vi "Plot_Uniform_Array.vi"(10 "Top Left Building Centre":sgl[](array[numeric])=[-1400.0, -945.0, 50.0] format="%#.2f") -> (0 "Status":T2)   [LabVIEW 2015]
uses:
  Anemometry Sub Vis/Gen Trav/Multi_Run_Status.ctl
  Anemometry Sub Vis/Controls/Tunnel_Coordinates.ctl
  Anemometry Sub Vis/Gen Trav/Traverse_cluster.ctl
  Anemometry Sub Vis/Gen Trav/Spacing.ctl
  Anemometry Sub Vis/Controls/Multi_run_mode.ctl
panel:
  in  "Work in Tunnel Coordinates?":T1
  out "Array":dbl[][](array[numeric])
  in  "Number of Columns":i32=8
  in  "Number of Rows":i32=21
  in  "dY Street":dbl=70.0
  in  "dX Street":dbl=70.0
  in  "dYBuilding":dbl=70.0
  in  "dX Building":dbl=140.0
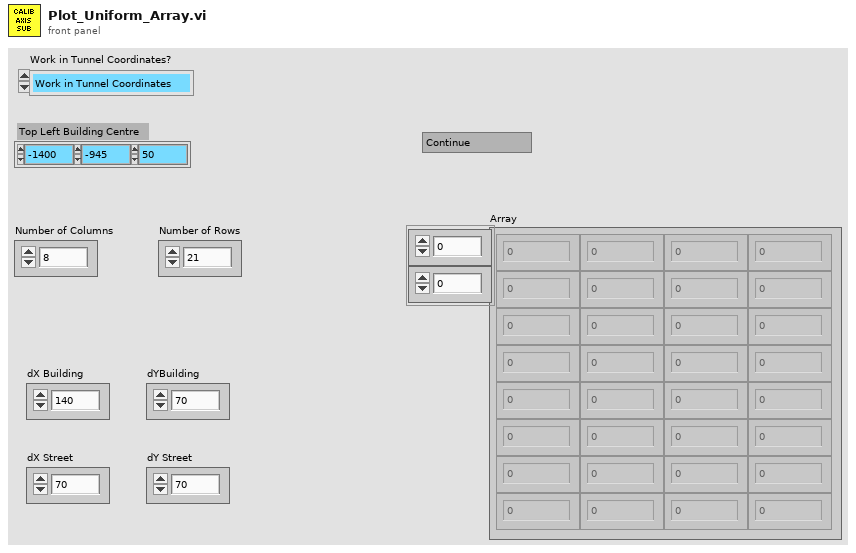
[diagram p1: front panel]
types:
  T1 = typedef "Tunnel_Coordinates.ctl" = enum16{"Work in Tunnel Coordinates", "Work in Model Coordinates"}
  T2 = typedef "Multi_Run_Status.ctl" = enum16{"Continue", "Jump to Next Point", "Jump to Next Row", "Jump To Fall Back", "Terminate Run"}
  T3 = typedef "Traverse_cluster.ctl" = cluster{"Start X":sgl, "Start Y":sgl, "Start Z":sgl, "End X":sgl, "End Y":sgl, "End Z":sgl, "No. of pts.":i32, "Spacing":T4, "Filename":path, "Tunnel Speed":dbl, "Averaging time (min)":dbl, "Extra Commands":string, "Carrier_1 Q (l/min)":dbl, "Carrier_2 Q (l/min)":dbl, "Trace Gas Concentration (%)":dbl, "Specific Arguments":string, "Comments":string, "Row No":i32, "Row Type Selector":T5, "Completion time":string, "Row Duration (mins)":dbl, "No. of Valid pts.":i32, "Meas Setup File":string}
  T4 = typedef "Spacing.ctl" = enum16{"Linear", "Log", "Gauss", "Specified", "N/A"}
  T5 = typedef "Multi_run_mode.ctl" = enum16{"Move Traverse Only", "Set Tunnel Speed Only", "Set Source Only", "Set Measurement Conditions", "Single Measurement", "Vertical Profile", "Lateral Profile", "Longitudinal Profile", "Explore Volume", "Multi-Axis Profile", "Auto Calibrate", "Meas Fast FID Bkgnd", "Check Beam Power", "Scanning Valve Measurement", "Run VI Named:", "Set ADAM Ch", "Wait (minutes)", "Send Message", "Synchronize With:", "Fall Back to this Row", "Turn Off Row Repeating", "Blank Row", "Traverse 3D Volume"}
  T6 = enum16{"Load Command File", "Save Command File", "Check Multi Run Prog", "Check Multi Run Prog With Live Moves", "Run Multi Run Prog"}
  T7 = enum16{"Load Command File", "Save Command File", "Check Multi Run Prog", "Check Multi Run Prog With Live Moves", "Run Multi Run Prog"}[]
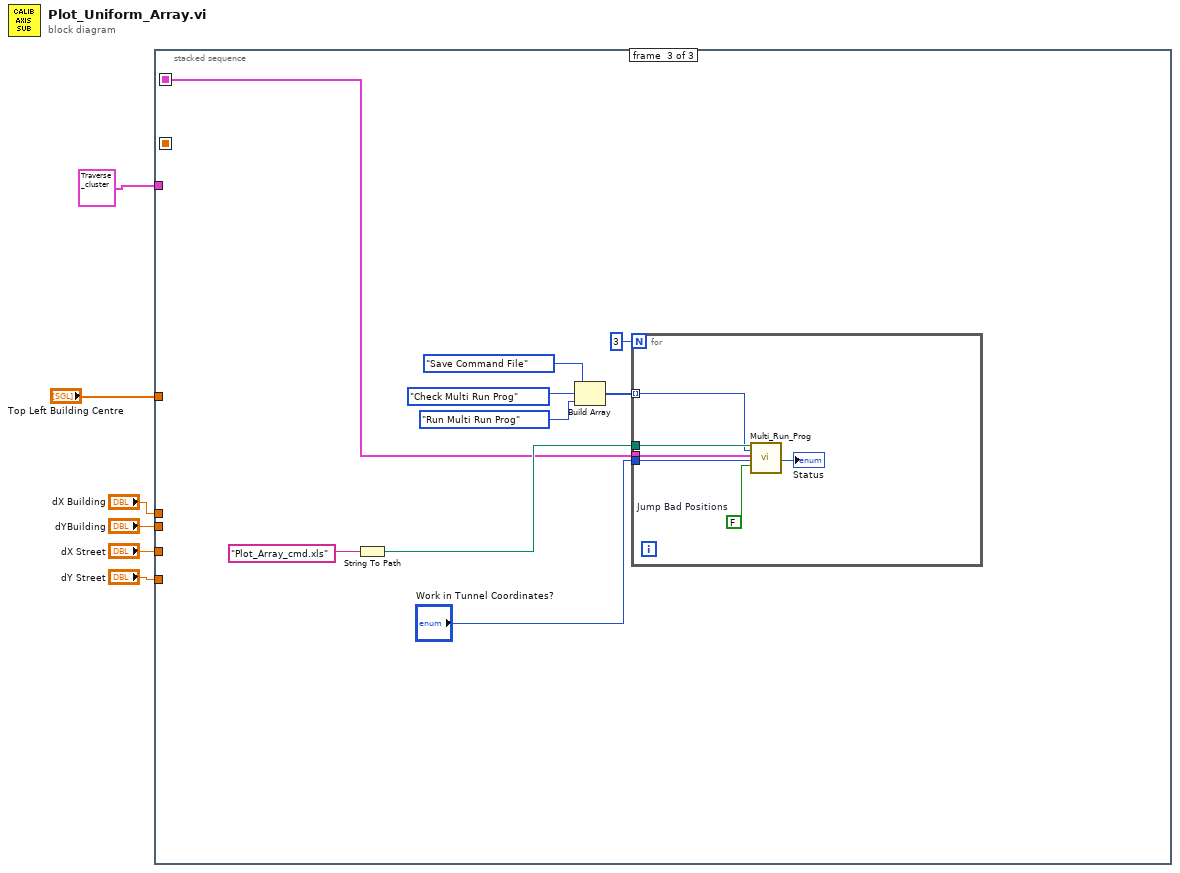
[diagram p0: block diagram]
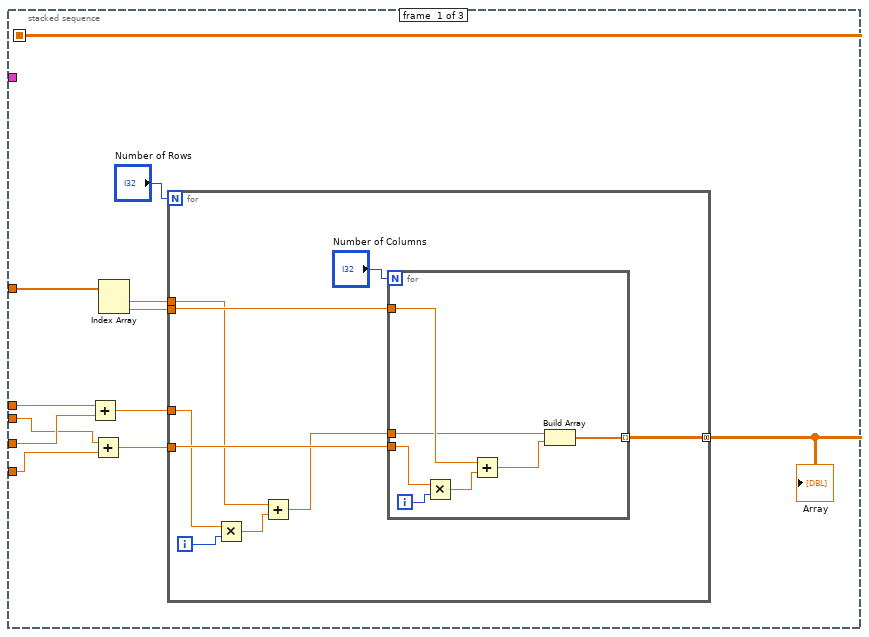
[diagram p2: hidden frame]
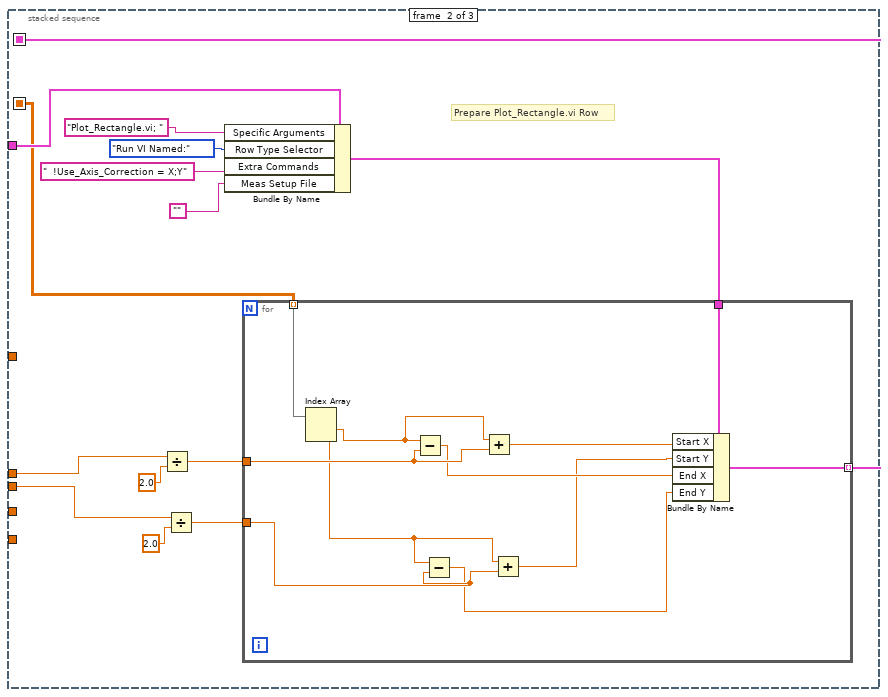
[diagram p3: hidden frame]
diagram:
  n1 = stacked-sequence {
    seq-local: [_ w35 _] -> [_ _ w62]
    seq-local: [w7 _ _] -> [_ w43 _]
    tunnel: "Top Left Building Centre" -> [w12 _ _]
    tunnel: T3 {"Start X"=2010.0, "Start Y"=1100.0, "Start Z"=50.0, "End X"=2010.0, "End Y"=-1300.0, "End Z"=50.0, "No. of pts."=49, "Spacing"=enum."Linear", "Filename"=path "E:/Enflo_Data_Local/2016/EnFlo_Tunnel/Paul_Hayden/Results/Res_04-2016/Y_Axis_Calibration_Y+100.xls", "Tunnel Speed"=0.0, "Averaging time (min)"=0.05, "Extra Commands"="!Datum Image = 50mm_Y_Strip.xls", "Carrier_1 Q (l/min)"=0.0, "Carrier_2 Q (l/min)"=0.0, "Trace Gas Concentration (%)"=0.0, "Specific Arguments"="Y= ;1100 ; 1050 ; 1000 ; 950 ; 900 ; 850 ; 800 ; 750 ; 700 ; 650 ; 600 ; 550 ; 500 ; 450 ; 400 ; 350 ; 300 ; 250 ; 200 ; 150 ; 100 ; 50 ; 0 ; -50 ; -100 ; -150 ; -200 ; -250 ; -300 ; -350 ; -400 ; -450 ; -500 ; -550 ; -600 ; -650 ; -700 ; -750 ; -800 ; -850 ; -900 ; -950 ; -1000 ; -1050 ; -1100 ; -1150 ; -1200 ; -1250 ; -1300 ; ", "Comments"="", "Row No"=1, "Row Type Selector"=enum."Lateral Profile", "Completion time"="10:16  04-04-2016", "Row Duration (mins)"=10.616666666666667, "No. of Valid pts."=49, "Meas Setup File"="Trav_Cam_Picture.xls"} ("Traverse line") -> [_ w46 _]
    tunnel: "dX Building" -> [w17 w42 _]
    tunnel: "dX Street" -> [w16 _ _]
    tunnel: "dYBuilding" -> [w15 w39 _]
    tunnel: "dY Street" -> [w14 _ _]
    frame #0 {
      n2 = Add(x=w17, y=w16) -> (x+y=w10:dbl)
      n3 = Add(x=w15, y=w14) -> (x+y=w13:dbl)
      n4 = Index Array(array=w12) -> (element #1=w9:sgl, element #2=w11:sgl)  [unwired: 2 in]
      n5 = for {
        N: "Number of Rows" -> [_]
        tunnel: w13 -> [w26]
        tunnel: w11 -> [w25]
        tunnel: w10 -> [w22]
        tunnel: w9 -> [w21]
        tunnel: [w18] -> w7 mode=concatenating
        i -> [w23]
        n6 = Multiply(x=w22, y=w23) -> (x*y=w24:dbl)
        n7 = Add(x=w21, y=w24) -> (x+y=w19:dbl)
        n8 = for {
          N: "Number of Columns" -> [_]
          tunnel: w26 -> [w32]
          tunnel: w25 -> [w30]
          tunnel: w19 -> [w29]
          tunnel: [w27] -> w18 mode=indexing
          i -> [w33]
          n9 = Multiply(x=w32, y=w33) -> (x*y=w31:dbl)
          n10 = Add(x=w30, y=w31) -> (x+y=w28:dbl)
          n11 = Build Array(w29, w28) -> (w27:dbl[])
        }
      }
      "Array" <- w7
    }
    frame #1 {
      # "Prepare Plot_Rectangle.vi Row"
      n12 = Divide(x=w42, y=2.0) -> (x/y=w38:dbl)
      n13 = Divide(x=w39, y=2.0) -> (x/y=w37:dbl)
      n14 = Bundle By Name(cluster=w46, "Specific Arguments"="Plot_Rectangle.vi; ", "Row Type Selector"=Multi_run_mode."Run VI Named:", "Extra Commands"="  !Use_Axis_Correction = X;Y", "Meas Setup File"="") -> (w36:T3)
      n15 = for {
        tunnel: w43 -> [w58] mode=indexing
        tunnel: w38 -> [w56]
        tunnel: w37 -> [w52]
        tunnel: w36 -> [w49]
        tunnel: [w48] -> w35 mode=indexing
        n16 = Index Array(array=w58) -> (element #1=w57:dbl, element #2=w53:dbl)  [unwired: 2 in]
        n17 = Subtract(x=w57, y=w56) -> (x-y=w54:dbl)
        n18 = Subtract(x=w53, y=w52) -> (x-y=w50:dbl)
        n19 = Add(x=w57, y=w56) -> (x+y=w55:dbl)
        n20 = Add(x=w53, y=w52) -> (x+y=w51:dbl)
        n21 = Bundle By Name(cluster=w49, "Start X"=w55, "Start Y"=w51, "End X"=w54, "End Y"=w50) -> (w48:T3)
      }
    }
    frame #2 {
      n22 = String To Path(string="Plot_Array_cmd.xls") -> (path=w67:path)
      n23 = Build Array(T6."Save Command File" ("Mode"), T6."Check Multi Run Prog" ("Mode"), T6."Run Multi Run Prog" ("Mode")) -> (w63:T7)
      n24 = for {
        N: 3 -> [_]
        tunnel: w62 -> [w73]
        tunnel: w67 -> [w72]
        tunnel: "Work in Tunnel Coordinates?" -> [w71]
        tunnel: w63 -> [w70] mode=indexing
        w69 = FALSE  # Jump Bad Positions
        n25 = call "Multi_Run_Prog.vi"("Command filename"=w72, "Mode"=w70, "Table"=w73, "Work in Tunnel Coordinates?"=w71, "Jump Bad Positions"=w69) -> ("Status"=→"Status":T2)  [unwired: 14 in]
      }
    }
  }
